vi "printDaqSignal.vi"(8 "error in":errorcluster, 9 "Indent":i32, 10 "TreeRef":refnum<vi>, 11 "baseObject in":refnum<class "IBaseObject.lvclass">) -> (0 "error out":errorcluster, 3 "baseObject out":refnum<class "IBaseObject.lvclass">)   [LabVIEW 2022 SP3, in "openDAQ.lvlib" / "daqUtils.lvlib" / "Tree.lvlib"]
uses:
  Tree.lvlib
  ISignal/ISignal.lvclass
  IBaseObject/IBaseObject.lvclass
  IBaseObject/Polymorphic/queryInterface/querySignalInterface.vi
  IComponent/IComponent.lvclass
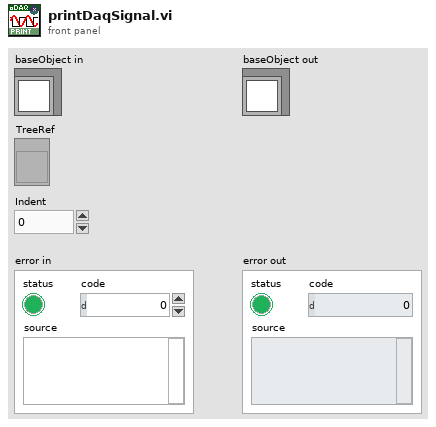
[diagram p1: front panel]
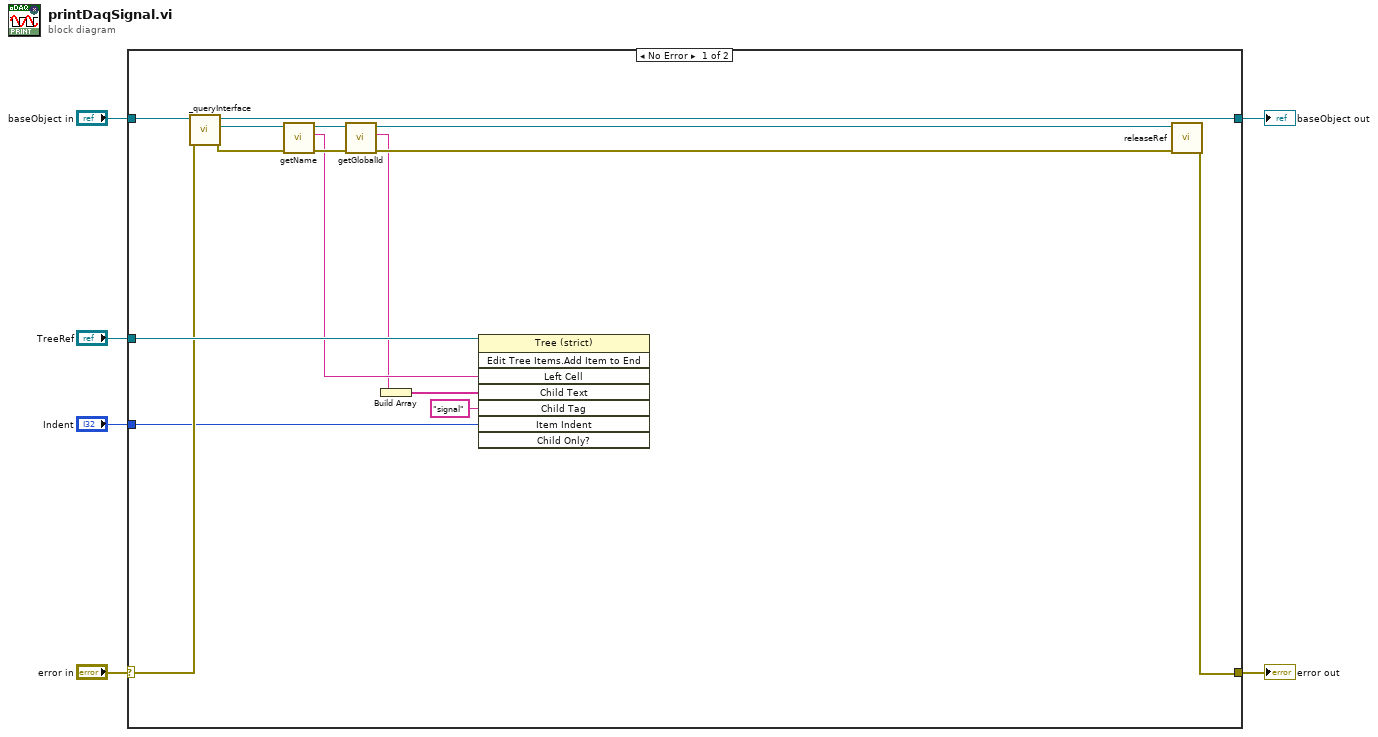
[diagram p0: block diagram]
diagram:
  n1 = case shown="No Error" "error in" {
    selector: "error in" -> [w16 w24]
    tunnel: "baseObject in" -> [w21 w23]
    tunnel: "Indent" -> [w14 _]
    tunnel: "TreeRef" -> [w17 _]
    tunnel: [w13 w24] -> w2
    tunnel: [w19 w23] -> w1
    frame No Error {
      n2 = call-poly "_queryInterface.vi"("error in (no error)"=w16, "IBaseObject in"=w21) -> ("error out"=w18:errorcluster, "ISignal out"=w20:refnum<class "ISignal.lvclass">, "IBaseObject out"=w19:refnum<class "IBaseObject.lvclass">)  [unwired: 7 in]
      n3 = call "getName.vi"("error in (no error)"=w18, "IComponent in"=w20) -> ("error out"=w22:errorcluster, "Name out"=w15:string, "IComponent out"=w11:refnum<class "ISignal.lvclass">)  [unwired: 7 in]
      n4 = call "getGlobalId.vi"("error in (no error)"=w22, "IComponent in"=w11) -> ("error out"=w9:errorcluster, "GlobalId out"=w8:string, "IComponent out"=w10:refnum<class "ISignal.lvclass">)  [unwired: 7 in]
      n5 = Build Array(w8) -> (w7:string[])
      n6 = invoke class="Tree (strict)" method="Edit Tree Items.Add Item to End"(reference=w17, "Left Cell"=w15, "Child Text"=w7, "Child Tag"="signal", "Item Indent"=w14) -> ()  [unwired: 3 in, 8 out]
      n7 = call-dynamic "releaseRef.vi"("error in (no error)"=w9, "IBaseObject in"=w10) -> ("error out"=w13:errorcluster)  [unwired: 9 in]
    }
    frame Error {
    }
  }
  "error out" <- w2
  "baseObject out" <- w1
